vi "Configure.vi"(8 "error in (no error)":errorcluster, 9 "Sample Frequency (100Hz)":T1(ring)=enum."100Hz", 10 "Accelerometer Sensitivity (1.5g)":enum8{"1.5g", "2g", "4g", "6g"}(ring), 11 "Sparkfun Atomic IMU in":refnum<class "Sparkfun Atomic IMU.lvclass">) -> (0 "error out":errorcluster, 3 "Sparkfun Atomic IMU out":refnum<class "Sparkfun Atomic IMU.lvclass">)   [LabVIEW 2019, in "Sparkfun Atomic IMU.lvclass"]
doc: "Configures sensor including accelerometer sensitivity, sensor sample frequency."
uses:
  Sparkfun Atomic IMU.lvclass
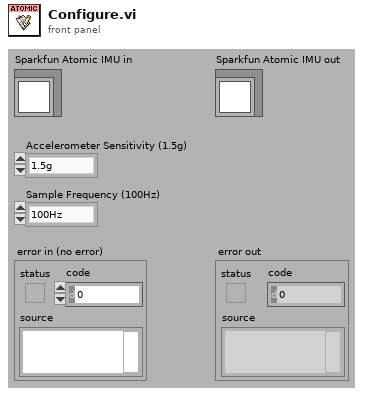
[diagram p1: front panel]
types:
  T1 = enum8{"50Hz", "100Hz", "150Hz", "200Hz", "250Hz"}
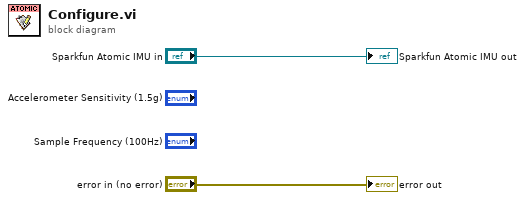
[diagram p0: block diagram]
diagram:
  "Sparkfun Atomic IMU out" <- "Sparkfun Atomic IMU in"
  "error out" <- "error in (no error)"
